vi "Update Pin Map from XML.vi"(8 "error in":errorcluster, 11 "request data":T2) -> (0 "error out":errorcluster, 3 "response data":T1)   [LabVIEW 2020, in "MeasurementLink TestStand Integration.lvlib"]
uses:
  MeasurementLink TestStand Integration.lvlib
  MeasurementLink Pin Map Client/RPC Messages/ni_measurementlink_pinmap_v1_UpdatePinMapFromXmlRequest.ctl
  MeasurementLink Pin Map Client/RPC Messages/ni_measurementlink_pinmap_v1_PinMap.ctl
  MeasurementLink gRPC Utilities/TypeDefs/Client Pool FGV Action.ctl
  MeasurementLink Pin Map Client/MeasurementLink Pin Map Client.lvlib
  MeasurementLink gRPC Utilities/MeasurementLink gRPC Utilities.lvlib
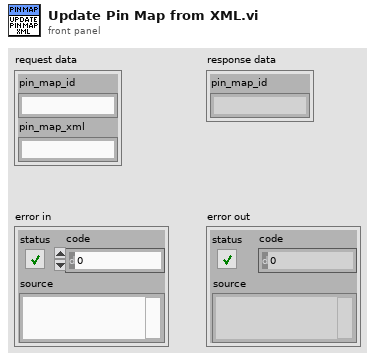
[diagram p1: front panel]
types:
  T1 = typedef "MeasurementLink Pin Map Client.lvlib/ni_measurementlink_pinmap_v1_PinMap.ctl" = cluster{"pin_map_id":string}
  T2 = typedef "MeasurementLink Pin Map Client.lvlib/ni_measurementlink_pinmap_v1_UpdatePinMapFromXmlRequest.ctl" = cluster{"pin_map_id":string, "pin_map_xml":string}
  T3 = typedef "MeasurementLink gRPC Utilities.lvlib/Client Pool FGV Action.ctl" = enum16{"Get Client", "Recreate Client"}
  T4 = typedef "grpc-lvsupport-release.lvlib/grpcId.ctl" = u64
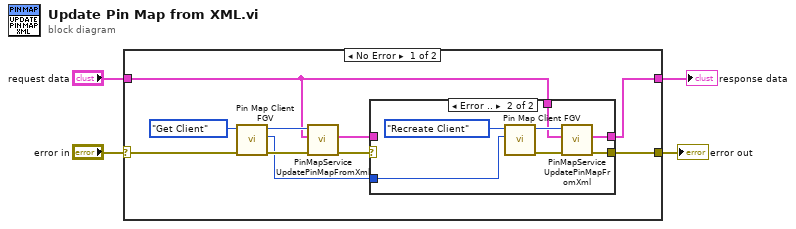
[diagram p0: block diagram]
diagram:
  n1 = case shown="No Error" "error in" {
    selector: "error in" -> [w14 w24]
    tunnel: [w10 w24] -> w3
    tunnel: "request data" -> [w5 _]
    tunnel: [w8 _] -> w1
    frame No Error {
      n2 = call "Pin Map Client FGV.vi"("error in"=w14, "action"=Client_Pool_FGV_Action."Get Client") -> ("error out"=w13:errorcluster, "unique id out"=w6:u64, "grpc client id"=w12:T4)  [unwired: 7 in]
      n3 = call "PinMapService UpdatePinMapFromXml.vi"("error in"=w13, "Request Data"=w5, "gRPC ID"=w12) -> ("error out"=w11:errorcluster, "Response Data"=w7:T1)  [unwired: 6 in, 1 out]
      n4 = case shown="Error .." w11 {
        selector: w11 -> [w16 _]
        tunnel: [w16 w20] -> w10
        tunnel: [w15 w19] -> w8
        tunnel: w7 -> [w15 _]
        tunnel: w6 -> [_ w18]
        tunnel: w5 -> [_ w17]
        frame No Error {
        }
        frame Error {
          n5 = call "Pin Map Client FGV.vi"("unique id in"=w18, "action"=Client_Pool_FGV_Action."Recreate Client") -> ("error out"=w21:errorcluster, "grpc client id"=w22:T4)  [unwired: 7 in, 1 out]
          n6 = call "PinMapService UpdatePinMapFromXml.vi"("error in"=w21, "Request Data"=w17, "gRPC ID"=w22) -> ("error out"=w20:errorcluster, "Response Data"=w19:T1)  [unwired: 6 in, 1 out]
        }
      }
    }
    frame Error {
    }
  }
  "error out" <- w3
  "response data" <- w1
